vi "File_Path Keeper.vi"(4 "Skip Dialogue":bool, 6 "DELETE":bool, 7 "OverWrite":bool, 8 "Error":errorcluster, 9 "INI File Path":path, 11 "File / Directory Name":string) -> (0 "Error Out":errorcluster, 2 "Valid Item Out":bool, 3 "Path Out":path=path "D:/Pitney PTS/PTS PROGRAMS/2-Sparks 1 and 2/SparksMain32.vi")   [LabVIEW 2020]
uses:
  <vilib>/Utility/config.llb/Read Key (Path).vi
  <vilib>/Utility/config.llb/NI_LVConfig.lvlib
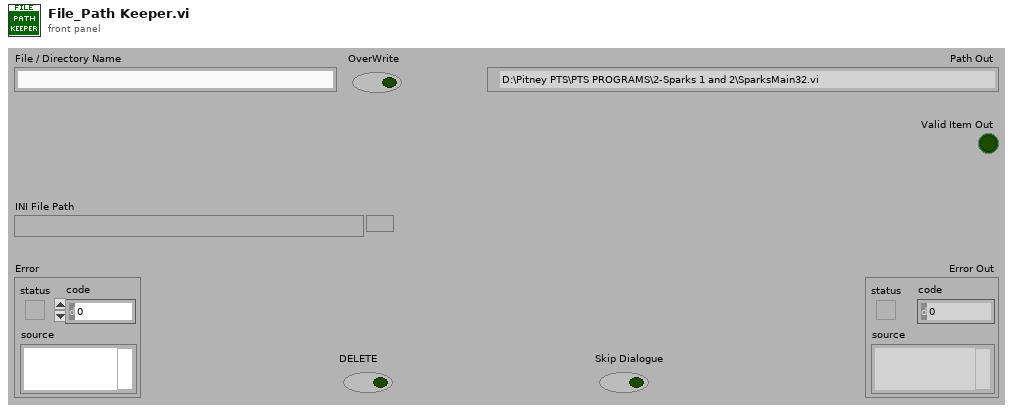
[diagram p1: front panel]
types:
  T1 = typedef "NI_LVConfig.lvlib/Config Data RefNum.ctl" = refnum<k1>
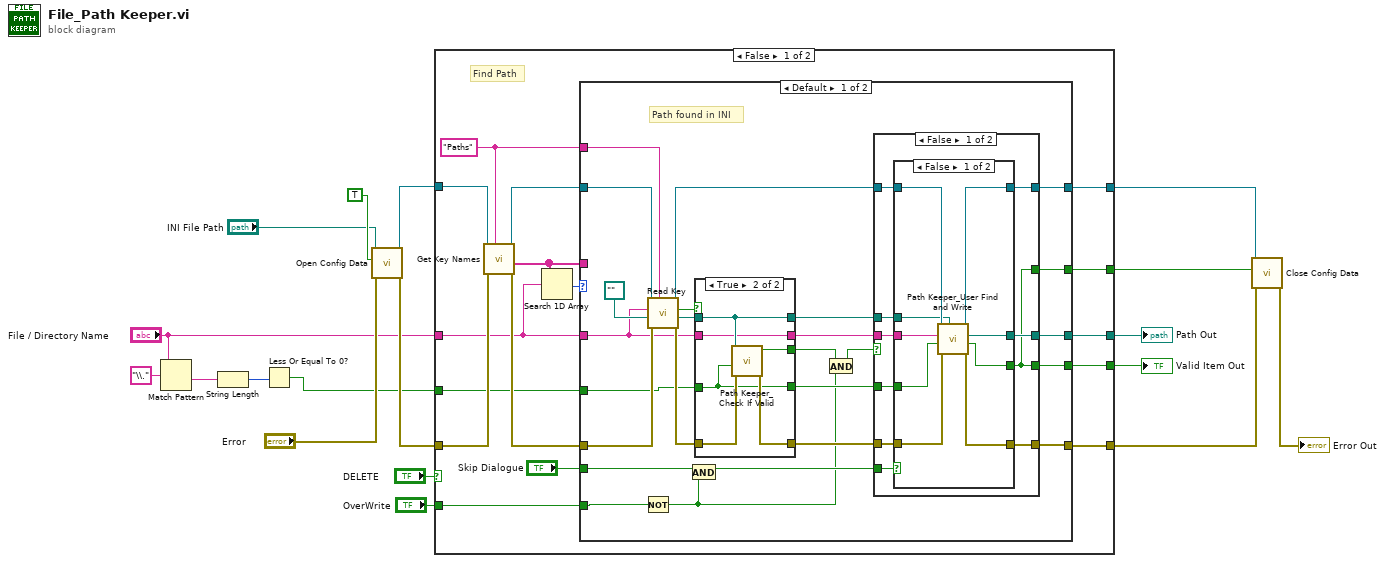
[diagram p0: block diagram]
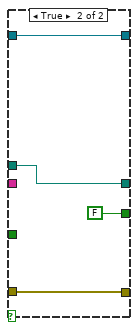
[diagram p2: hidden frame]
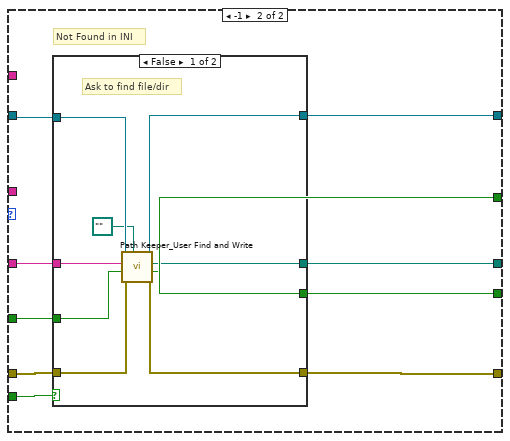
[diagram p5: hidden frame]
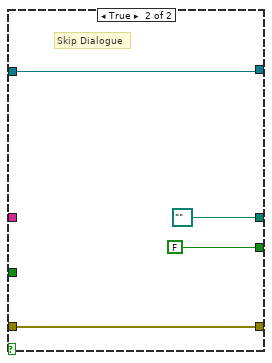
[diagram p6: hidden frame]
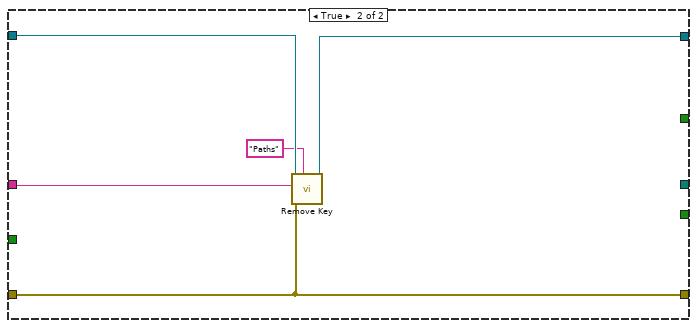
[diagram p7: hidden frame]
diagram:
  n1 = Match Pattern(string="File / Directory Name", regular expression="\\.") -> (after substring=w4:string)  [unwired: 1 in, 3 out]
  n2 = String Length(string=w4) -> (length=w3:i32)
  n3 = Less Or Equal To 0?(x=w3) -> (x <= 0?=w2:bool)
  n4 = call <vilib>:"Open Config Data.vi"("error in (no error)"="Error", "create file if necessary (T)"=TRUE ("create file if necessary? (T)"), "configuration file path"="INI File Path") -> ("error out"=w12:errorcluster, "refnum"=w13:T1)  [unwired: 6 in, 1 out]
  n5 = case shown="False" "DELETE" {
    tunnel: [w34 w120] -> w18
    tunnel: [w33 w122] -> w16
    tunnel: w13 -> [w32 w121]
    tunnel: w12 -> [w30 w122]
    tunnel: "File / Directory Name" -> [w27 w123]
    tunnel: [w24 _] -> w11
    tunnel: [w23 _] -> w10
    tunnel: [w22 _] -> w8
    tunnel: w2 -> [w21 _]
    tunnel: "OverWrite" -> [w19 _]
    frame False {
      w25 = "Paths" ("section")
      # "Find Path"
      n6 = call <vilib>:"Get Key Names.vi"("section"=w25, "error in (no error)"=w30, "refnum"=w32) -> ("error out"=w29:errorcluster, "key names"=w28:string[], "refnum out"=w31:T1)  [unwired: 5 in, 1 out]
      n7 = Search 1D Array(1D array=w28, element=w27) -> (index of element=w26:i32)  [unwired: 1 in]
      n8 = case shown="Default" w26 {
        tunnel: w31 -> [w59 w104]
        tunnel: w27 -> [w42 w100]
        tunnel: [w48 w101] -> w34
        tunnel: [w51 w102] -> w33
        tunnel: w29 -> [w57 w103]
        tunnel: w28 -> [_ _]
        tunnel: w21 -> [w52 w105]
        tunnel: w25 -> [w58 _]
        tunnel: [w46 w99] -> w24
        tunnel: [w45 w98] -> w22
        tunnel: [w41 w98] -> w23
        tunnel: "Skip Dialogue" -> [w40 w97]
        tunnel: w19 -> [w39 _]
        frame Default {
          # "Path found in INI"
          n9 = Not(x=w39) -> (.not. x?=w37:bool)
          n10 = call-poly <vilib>:"Read Key.vi"("section"=w58, "error in (no error)"=w57, "default value"=path "", "key"=w42, "refnum"=w59) -> ("error out"=w55:errorcluster, "value"=w53:path, "found?"=w54:bool, "refnum out"=w49:T1)  [unwired: 3 in]
          n11 = And(x=w40, y=w37) -> (x .and. y?=w38:bool)
          n12 = case shown="True" w54 {
            tunnel: w55 -> [w89 w96]
            tunnel: [w89 w95] -> w50
            tunnel: w53 -> [w90 w93]
            tunnel: w52 -> [w88 w92]
            tunnel: [_ w94] -> w35
            tunnel: [w90 w93] -> w47
            tunnel: [w88 w92] -> w44
            tunnel: [w87 w91] -> w43
            tunnel: w42 -> [w87 w91]
            frame False {
            }
            frame True {
              n13 = call "Path Keeper_Check If Valid.vi"("error In"=w96, "File(f)\nDirectory(t) In"=w92, "path In"=w93) -> ("error Out"=w95:errorcluster, "Valid Out"=w94:bool)  [unwired: 7 in]
            }
          }
          n14 = And(x=w35, y=w37) -> (x .and. y?=w36:bool)
          n15 = case shown="False" w36 {
            selector: w36 -> [_ w83]
            tunnel: [w69 w85] -> w51
            tunnel: w50 -> [w68 w85]
            tunnel: w49 -> [w67 w84]
            tunnel: [w66 w84] -> w48
            tunnel: [w65 w86] -> w46
            tunnel: w47 -> [w61 w86]
            tunnel: [w62 w83] -> w45
            tunnel: w43 -> [w64 _]
            tunnel: w44 -> [w63 _]
            tunnel: [w62 _] -> w41
            tunnel: w38 -> [w60 _]
            frame False {
              n16 = case shown="False" w60 {
                tunnel: [w78 w80] -> w69
                tunnel: w68 -> [w77 w80]
                tunnel: w67 -> [w76 w82]
                tunnel: [w75 w82] -> w66
                tunnel: [w74 w81] -> w65
                tunnel: w64 -> [w73 _]
                tunnel: w63 -> [w72 _]
                tunnel: [w71 FALSE ("Valid Path Out")] -> w62
                tunnel: w61 -> [w70 w81]
                frame False {
                  n17 = call "Path Keeper_User Find and Write.vi"("Previous location"=w70, "Error In"=w77, "File(f)\nDirectory(t) In"=w72, "File / Directory Name In"=w73, "Refnum In"=w76) -> ("Error Out"=w78:errorcluster, "Valid Path Out"=w71:bool, "Path Out"=w74:path, "Config Data Out"=w75:T1)  [unwired: 3 in]
                }
                frame True {
                }
              }
            }
            frame True {
            }
          }
        }
        frame -1 {
          # "Not Found in INI"
          n18 = case shown="False" w97 {
            tunnel: w105 -> [w114 _]
            tunnel: w104 -> [w113 w118]
            tunnel: w103 -> [w112 w115]
            tunnel: [w111 w115] -> w102
            tunnel: [w110 w118] -> w101
            tunnel: w100 -> [w109 _]
            tunnel: [w108 path "" ("Path Out")] -> w99
            tunnel: [w107 FALSE ("Valid Path Out")] -> w98
            frame False {
              # "Ask to find file/dir"
              n19 = call "Path Keeper_User Find and Write.vi"("Previous location"=path "", "Error In"=w112, "File(f)\nDirectory(t) In"=w114, "File / Directory Name In"=w109, "Refnum In"=w113) -> ("Error Out"=w111:errorcluster, "Valid Path Out"=w107:bool, "Path Out"=w108:path, "Config Data Out"=w110:T1)  [unwired: 3 in]
            }
            frame True {
              # "Skip Dialogue"
            }
          }
        }
      }
    }
    frame True {
      n20 = call <vilib>:"Remove Key.vi"("section"="Paths", "error in (no error)"=w122, "key"=w123, "refnum"=w121) -> ("refnum out"=w120:T1)  [unwired: 5 in, 2 out]
    }
  }
  "Path Out" <- w11
  "Valid Item Out" <- w8
  n21 = call <vilib>:"Close Config Data.vi"("error in (no error)"=w16, "write file if changed (T)"=w10, "refnum"=w18) -> ("error out"=→"Error Out":errorcluster)  [unwired: 7 in, 1 out]
